vi "Telegram Date to TimeStamp.vi"(11 "date":i64) -> (3 "time stamp":timestamp)   [LabVIEW 2015, in "Telegram Library.lvlib"]
doc: "Created IvanLis by LabVIEW Portal\nProfile: http://labviewportal.org/memberlist.php?mode=viewprofile&u=987\neMail: IvanLisanov@gMail.com\nTelegram: https://t.me/IvanLis"
uses:
  Telegram Library.lvlib
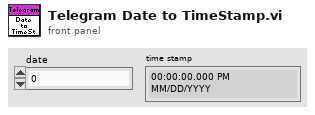
[diagram p1: front panel]
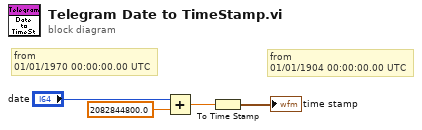
[diagram p0: block diagram]
diagram:
  # "from\n01/01/1904 00:00:00.00 UTC"
  # "from\n01/01/1970 00:00:00.00 UTC"
  n1 = Add(x="date", y=2082844800.0) -> (x+y=w2:dbl)
  n2 = To Time Stamp(1:w2) -> (0:→"time stamp":timestamp)
